vi "gantry_microcontroller_read_clockrate.vi"(11 "read inc/dec motor speed":string) -> (0 "number":i32)   [LabVIEW 2021]
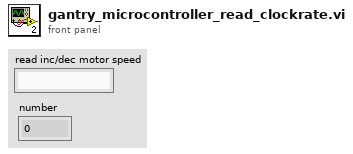
[diagram p1: front panel]
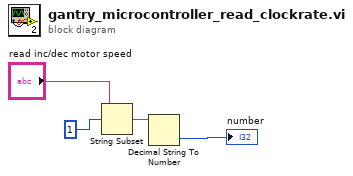
[diagram p0: block diagram]
diagram:
  n1 = String Subset(string="read inc/dec motor speed", offset (0)=1) -> (substring=w3:string)  [unwired: 1 in]
  n2 = Decimal String To Number(string=w3) -> (number=→"number":i32)  [unwired: 2 in, 1 out]
